vi "StartRunningCurrentProtocol.vi"   [LabVIEW 2018]
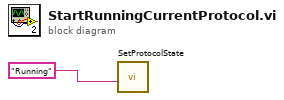
[diagram p0: block diagram]
diagram:
  n1 = call "SetProtocolState.vi"("state"="Running") -> ()  [unwired: 11 in]
